vi "Create and Add Instrument.vi"(6 "Physical Instr CFGs":string[](array[string]), 8 "error in":errorcluster, 11 "Target MSS in":refnum<class "CRIO MSS Test Actor.lvclass">) -> (0 "error out":errorcluster, 3 "Target MSS out":refnum<class "CRIO MSS Test Actor.lvclass">)   [LabVIEW 2023, in "CRIO MSS Test Actor.lvlib" / "CRIO MSS Test Actor.lvclass"]
uses:
  CRIO MSS Test Actor.lvclass
  CRIO MSS Test Actor.lvclass/CRIO MSS Test Actor.ctl
  Target Measure and Stimulus Subsystems/Target Measure and Stimulus Subsystems.lvclass
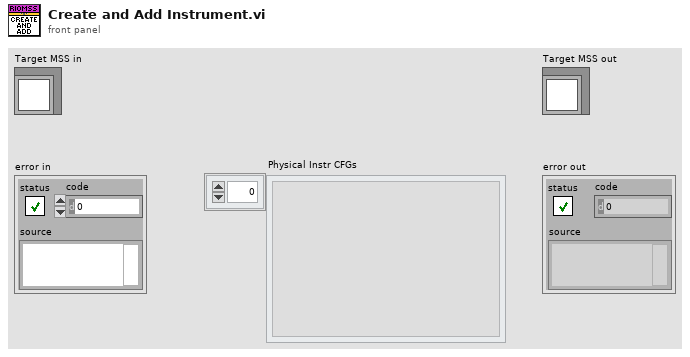
[diagram p1: front panel]
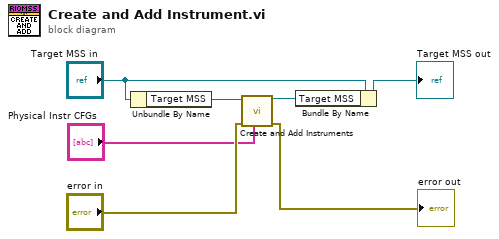
[diagram p0: block diagram]
diagram:
  n1 = Unbundle By Name("Target MSS in") -> ("Target MSS"=w6:refnum<class "Target Measure and Stimulus Subsystems.lvclass">)
  n2 = call-dynamic "Create and Add Instruments.vi"("Physical Instr CFGs"="Physical Instr CFGs", "Error In"="error in", "Target Measure and Stimulus Subsystems in"=w6) -> ("Error Out"=→"error out":errorcluster, "Target Measure and Stimulus Subsystems out"=w2:refnum<class "Target Measure and Stimulus Subsystems.lvclass">)  [unwired: 7 in]
  n3 = Bundle By Name(cluster="Target MSS in", "Target MSS"=w2) -> (→"Target MSS out":refnum<class "CRIO MSS Test Actor.lvclass">)
